vi "AREA DEL TRIANGULO P.APLICADA.vi"() -> ()   [LabVIEW 2020]
panel:
  in  "ALTURA":dbl
  in  "BASE":dbl
  out "AREA DEL TRIANGULO":dbl
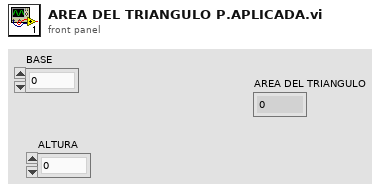
[diagram p1: front panel]
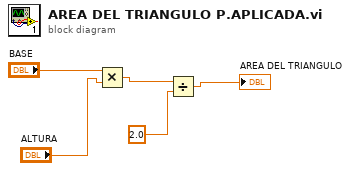
[diagram p0: block diagram]
diagram:
  n1 = Multiply(x="BASE", y="ALTURA") -> (x*y=w3:dbl)
  n2 = Divide(x=w3, y=2.0) -> (x/y=→"AREA DEL TRIANGULO":dbl)
